vi "Separacion Mensaje.vi"(11 "Mensaje":string) -> (0 "Z":string, 1 "Y":string, 2 "X":string, 3 "Arreglo Entradas":string[](array[string]))   [LabVIEW 2013, in "Proyecto 2 Touch.lvrbt"]
uses:
  Proyecto 2 Touch.lvrbt
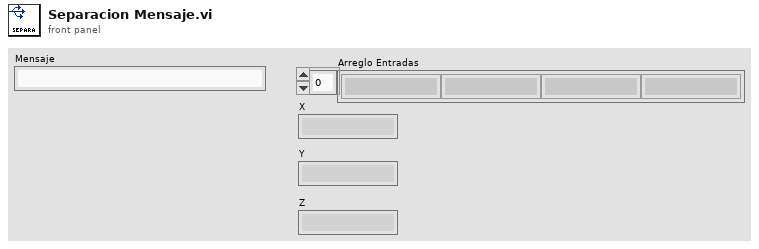
[diagram p1: front panel]
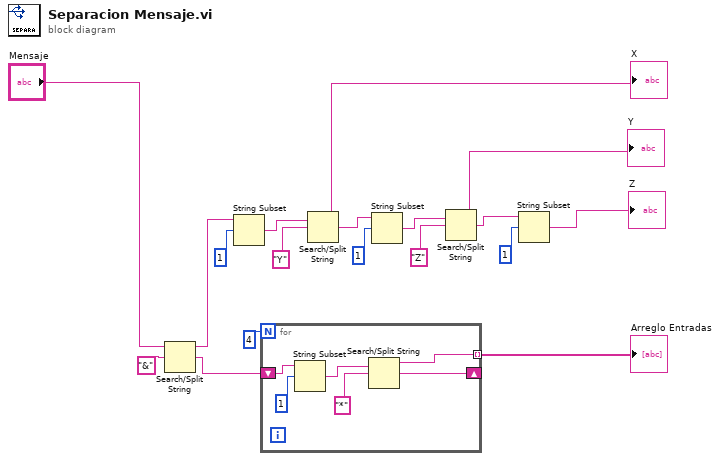
[diagram p0: block diagram]
diagram:
  n1 = Search/Split String(string="Mensaje", search string/char (-)="&") -> (substring before match=w10:string, match + rest of string=w16:string)  [unwired: 1 in, 1 out]
  n2 = String Subset(string=w10, offset (0)=1) -> (substring=w12:string)  [unwired: 1 in]
  n3 = for {
    N: 4 -> [_]
    tunnel: [w20] -> w14 mode=indexing
    shift-right: [w19] -> _
    shift-left: w16 -> [w23]
    n4 = String Subset(string=w23, offset (0)=1) -> (substring=w22:string)  [unwired: 1 in]
    n5 = Search/Split String(string=w22, search string/char (-)="*") -> (substring before match=w20:string, match + rest of string=w19:string)  [unwired: 1 in, 1 out]
  }
  "Arreglo Entradas" <- w14
  n6 = Search/Split String(string=w12, search string/char (-)="Y") -> (substring before match=→"X":string, match + rest of string=w3:string)  [unwired: 1 in, 1 out]
  n7 = String Subset(string=w3, offset (0)=1) -> (substring=w8:string)  [unwired: 1 in]
  n8 = Search/Split String(string=w8, search string/char (-)="Z") -> (substring before match=→"Y":string, match + rest of string=w5:string)  [unwired: 1 in, 1 out]
  n9 = String Subset(string=w5, offset (0)=1) -> (substring=→"Z":string)  [unwired: 1 in]
